vi "4-7 PrimeNumber.vi"() -> ()   [LabVIEW 2014]
doc: "------------------------------------\nAuther: Koji Ohashi\nModified: Hirotake Watashima\nCopyright (c) 2020 Japan LabVIEW Users Group, Volunteer members.\nThis VI is released under the MIT License.\nhttp://opensource.org/licenses/mit-license.php\n------------------------------------"
panel:
  out "size(s)":i32
  out "Prime Numbers":i32[](array[numeric])
  in  "N:Search upper limit (N>2)":i32=10000 min=3 step=1
  # "List of prime numbers\nby Elastotels sieve"
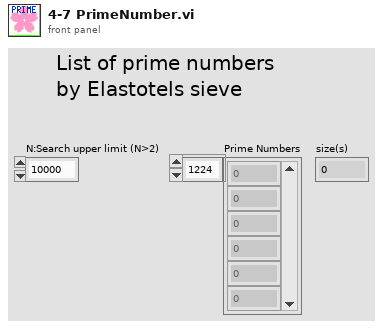
[diagram p1: front panel]
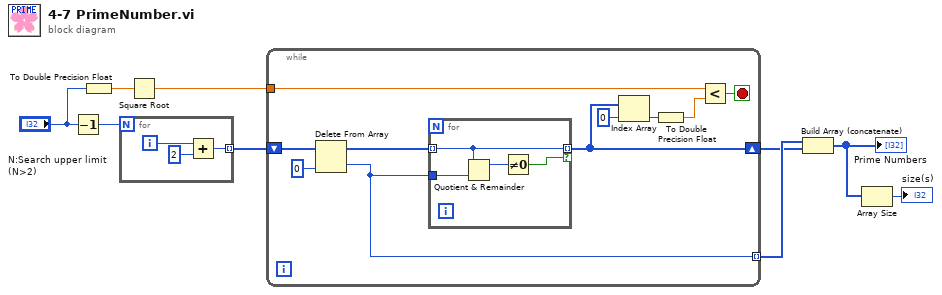
[diagram p0: block diagram]
diagram:
  n1 = Decrement(x="N:Search upper limit (N>2)") -> (x-1=w7:i32)
  n2 = To Double Precision Float(number="N:Search upper limit (N>2)") -> (double precision float=w2:dbl)
  n3 = for {
    N: w7 -> [_]
    tunnel: [w10] -> w1 mode=indexing
    i -> [w11]
    n4 = Add(x=w11, y=2) -> (x+y=w10:i32)
  }
  n5 = Square Root(x=w2) -> (sqrt(x)=w3:dbl)
  n6 = while {
    shift-right: [w21] -> w8
    shift-left: w1 -> [w22]
    tunnel: w3 -> [w18]
    tunnel: [w14] -> w9 mode=indexing
    stop <- w17 stop-if-true
    n7 = Delete From Array "Delete From Array"(array=w22, index=0 ("指標")) -> (deleted portion=w14:i32, array with subset deleted=w15:i32[])  [unwired: 1 in]
    n8 = for {
      tunnel: w15 -> [w24] mode=indexing
      tunnel: w14 -> [w26]
      tunnel: [w24] -> w21 mode=indexing if=w23
      n9 = Quotient & Remainder(x=w24, y=w26) -> (x-y*floor(x/y)=w25:i32)  [unwired: 1 out]
      n10 = Not Equal To 0?(x=w25) -> (x != 0?=w23:bool)
    }
    n11 = Index Array "Index Array"(array=w21, index=0) -> (element=w19:i32)
    n12 = To Double Precision Float(number=w19) -> (double precision float=w16:dbl)
    n13 = Less?(x=w18, y=w16) -> (x < y?=w17:bool)
  }
  n14 = Build Array (concatenate) "Build Array"(w9, w8) -> (w5:i32[])
  "Prime Numbers" <- w5
  n15 = Array Size(array=w5) -> (size(s)=→"size(s)":i32)
